vi "EJEM7.vi"() -> ()   [LabVIEW 2013]
panel:
  out "Waveform Graph":cluster{dbl, i32, i32[]}[](graph)
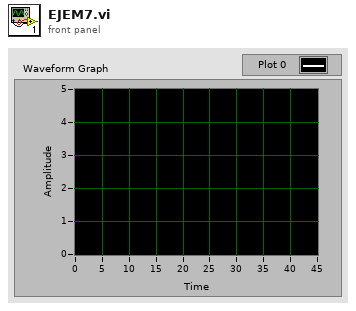
[diagram p1: front panel]
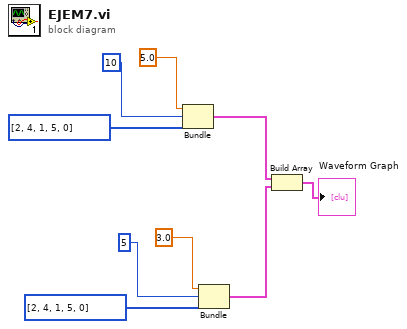
[diagram p0: block diagram]
diagram:
  n1 = Bundle(5.0, 10, i32[] [2, 4, 1, 5, 0]) -> (w3:cluster{dbl, i32, i32[]})  [unwired: 1 in]
  n2 = Bundle(3.0, 5, i32[] [2, 4, 1, 5, 0]) -> (w2:cluster{dbl, i32, i32[]})  [unwired: 1 in]
  n3 = Build Array(w3, w2) -> (→"Waveform Graph":cluster{dbl, i32, i32[]}[])
